vi "ConvertVtodBm.vi"(4 "voltage":dbl) -> (1 "dBm":dbl)   [LabVIEW 2017]
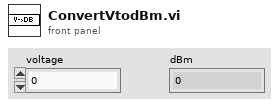
[diagram p1: front panel]
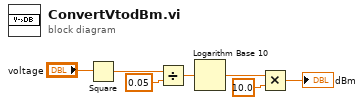
[diagram p0: block diagram]
diagram:
  n1 = Square(x="voltage") -> (x^2=w7:dbl)
  n2 = Divide(x=w7, y=0.05) -> (x/y=w5:dbl)
  n3 = Logarithm Base 10(1:w5) -> (0:w4:dbl)
  n4 = Multiply(x=w4, y=10.0) -> (x*y=→"dBm":dbl)
